vi "AcqErrorMessageTlog.vi"() -> ()   [LabVIEW 2010]
uses:
  <vilib>/Utility/error.llb/ErrWarn.ctl
  <vilib>/Utility/error.llb/DialogType.ctl
  <userlib>/TLogger/AcqErrorGlobalTlog.vi
panel:
  out "Error or Warning Glyph":T1=TRUE
  in  "stop":bool
  out "message":string=" INSTRUCTIONS:\r\rNormal Use:  When using subVIs that incorporate the error in/error out (or error I/O) structure, place this handler where you want to inform the user of an error, typically at the end of the I/O data path, as the last action of the program.  If the error in error? is ERROR, the handler creates a message describing the error and its source.  If the type of dialog = 1 (default), the message is displayed to the user, who can only acknowedge it.  If the type = 2, the user can acknowledge the message or abort execution; aborting a program with active I/O is not recommended.  If the type = 0, no message is displayed; this is used to process the error programmatically, and the error out cluster elements are wired to individual terminals for that reason.  \r\rOther Use:\n\r\nlocal testing.  To test the error code of a subVI or function that does not have the error I/O structure, you can wire its error code and a source string to the local error code and error source inputs.  If error in error? indicates no error and error code is not equal to 0, the local code and source are substituted for the error in values, and error? is set TRUE (ERROR)."
  out "error out":errorcluster
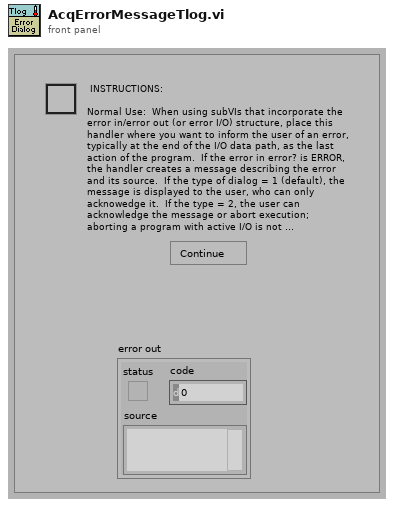
[diagram p1: front panel]
types:
  T1 = typedef "ErrWarn.ctl" = bool
  T2 = typedef "DialogType.ctl" = u16
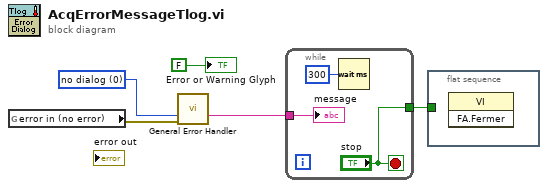
[diagram p0: block diagram]
diagram:
  w5 = T2 0 items=["no dialog", "OK message", "continue or stop message", "OK message + warnings", "continue/stop + warnings"] ("type of dialog (OK msg:1)")
  n1 = global read "AcqErrorGlobalTlog.vi" "error in (no error)"() -> (w4:errorcluster)
  n2 = call <vilib>:"General Error Handler.vi"("type of dialog (OK msg:1)"=w5, "error in (no error)"=w4) -> ("message"=w3:string)  [unwired: 9 in, 4 out]
  n3 = while {
    tunnel: w3 -> [w8]
    tunnel: ["stop"] -> w1
    stop <- "stop" stop-if-true
    n4 = Wait (ms)(milliseconds to wait=u32 300) -> ()  [unwired: 1 out]
    "message" <- w8
  }
  n5 = flat-sequence {
    tunnel: w1 -> [_]
    frame #0 {
      n6 = invoke class="VI" method="FA.Fermer"() -> ()  [unwired: 3 in, 3 out]
    }
  }
  "Error or Warning Glyph" <- T1 FALSE ("Error or Warning Glyph")
